vi "Initialize.vi"(7 "Channel Name":string="Setpoint.ch%d.SP", 8 "error in":errorcluster, 9 "Number of Channels":u32=1, 10 "Instance Name":string="PluginName", 11 "Voltage Limit in":refnum<class "Voltage Limit.lvclass">) -> (0 "error out":errorcluster caption="error in", 2 "Channel":T1[](array[typedef]), 3 "Voltage Limit out":refnum<class "Voltage Limit.lvclass">)   [LabVIEW 2023, in "Voltage Limit.lvclass"]
uses:
  Voltage Limit.lvclass
  Parents/Limit/Limit.lvclass
  Utilities/Channel.ctl
  Utilities/Utilities.lvlib
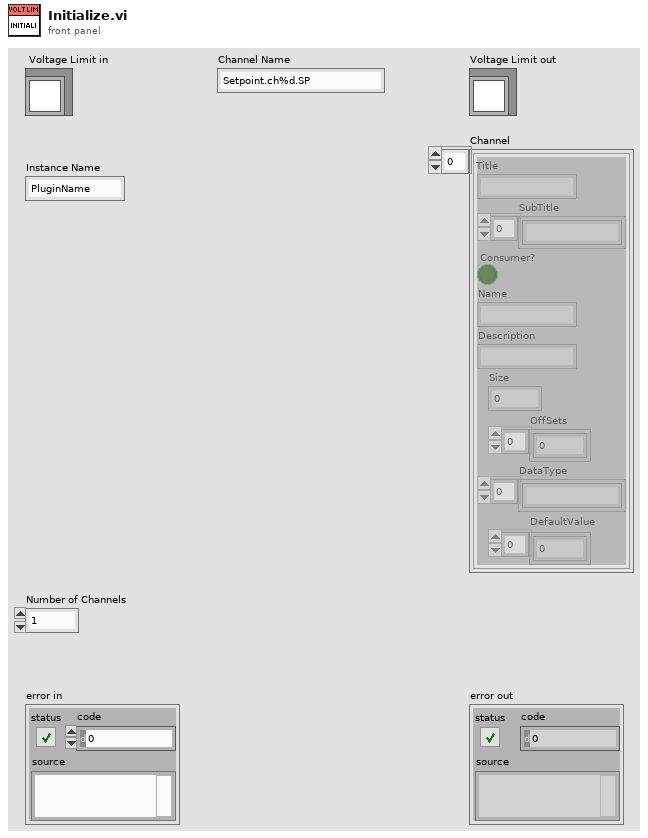
[diagram p1: front panel]
types:
  T1 = typedef "Utilities.lvlib/Channel.ctl" = cluster{"Title":string, "SubTitle":string[], "Consumer?":bool, "Name":string, "Description":string, "Size":i32, "OffSets":i32[], "DataType":string[], "DefaultValue":dbl[]}
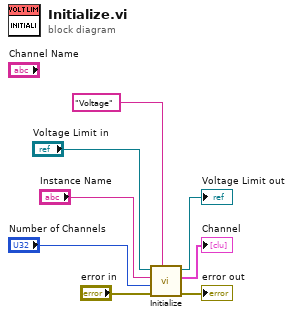
[diagram p0: block diagram]
diagram:
  n1 = call-parent "Initialize.vi"("Limit Name"="Voltage" ("LimitMAX.ch%d.SP"), "error in"="error in", "Number of Channels"="Number of Channels", "Instance Name"="Instance Name", "Limit in"="Voltage Limit in") -> ("error out"=→"error out":errorcluster, "Channel"=→"Channel":T1[], "Limit out"=→"Voltage Limit out":refnum<class "Voltage Limit.lvclass">)  [unwired: 4 in]
